vi "LockOut.vi"() -> ()   [LabVIEW 2019]
uses:
  <vilib>/NI/AMC/Read Termination Message.vi
  <vilib>/NI/AMC/Create Single Message.vi
  <vilib>/NI/AMC/Update Message Routing Info.vi
  <vilib>/NI/AMC/Globals.vi
  <vilib>/NI/AMC/Send Message.vi
  <vilib>/NI/AMC/AMC.lvlib
panel:
  out "By Emp:":string
  out "status":string
  in  "exit":bool
  # "Machine Locked Out"
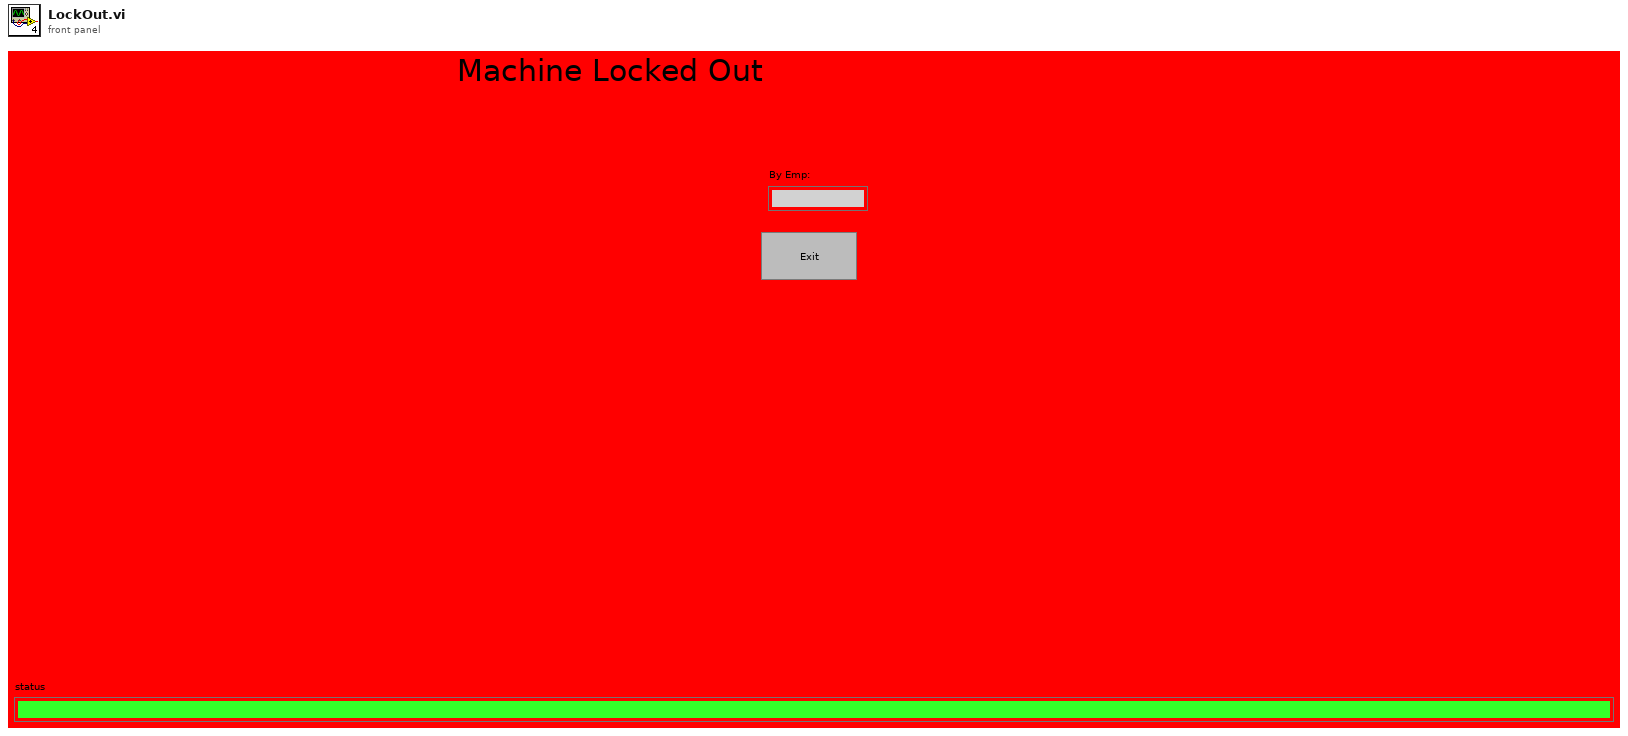
[diagram p1: front panel]
types:
  T1 = typedef "AMC.lvlib/Message Queue.ctl" = refnum<queue>
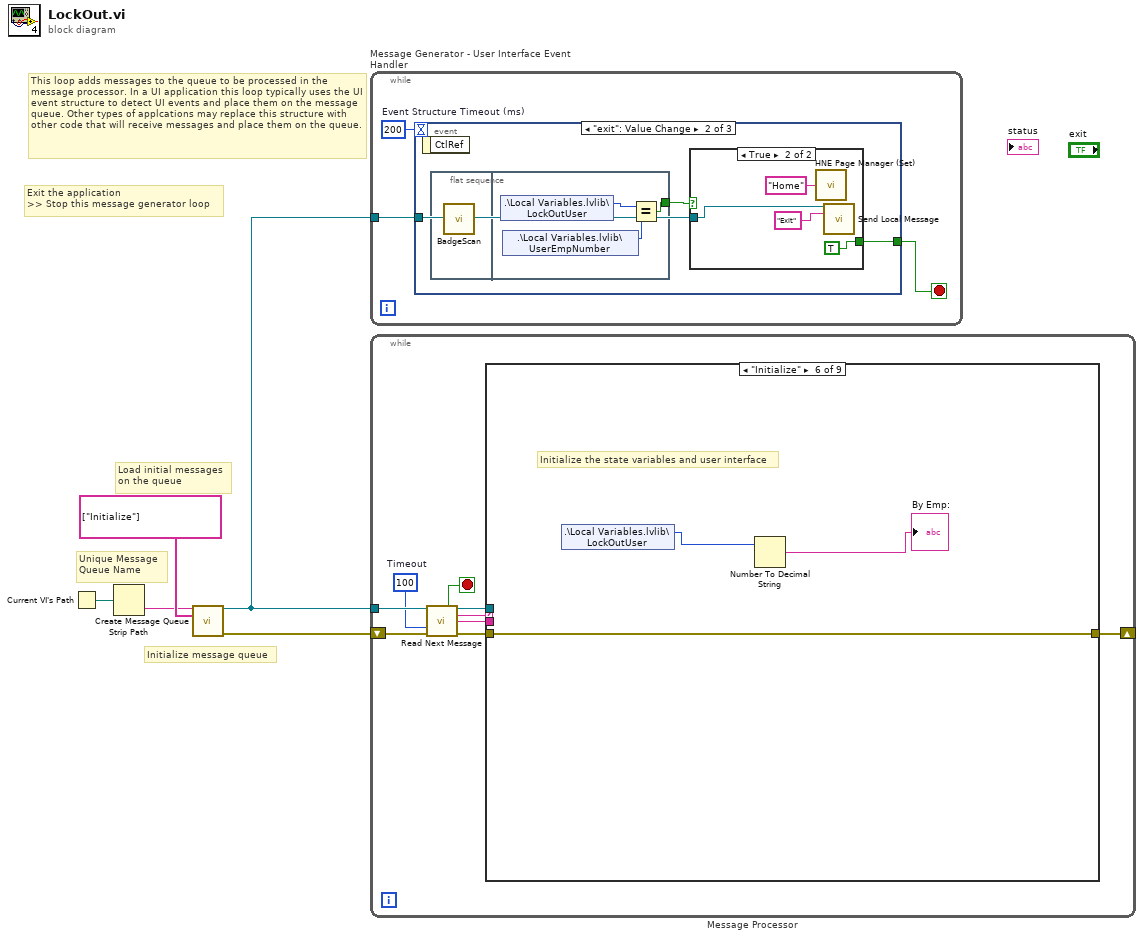
[diagram p0: block diagram]
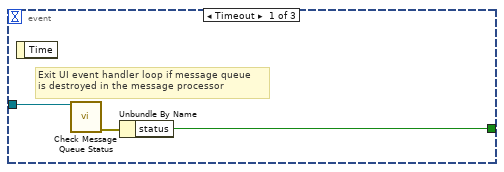
[diagram p2: hidden frame]
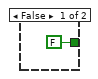
[diagram p3: hidden frame]
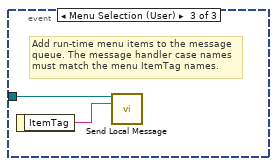
[diagram p4: hidden frame]
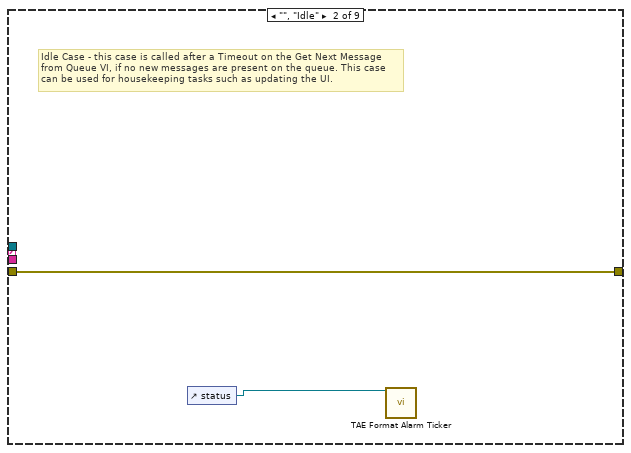
[diagram p6: hidden frame]
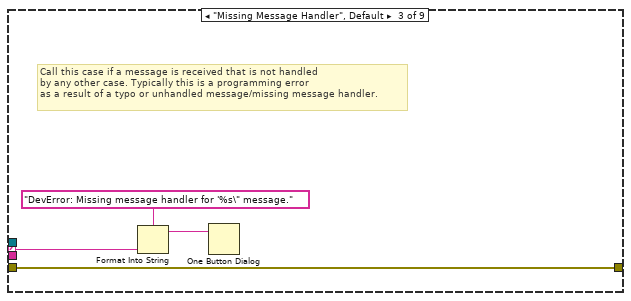
[diagram p7: hidden frame]
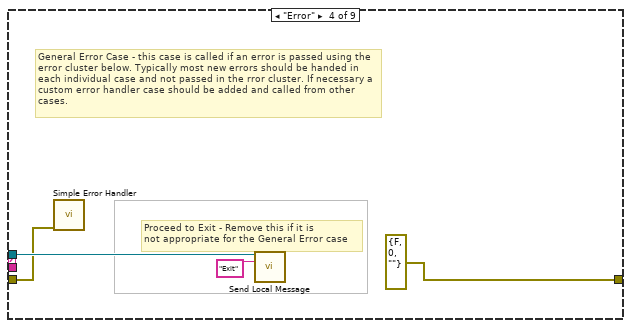
[diagram p8: hidden frame]
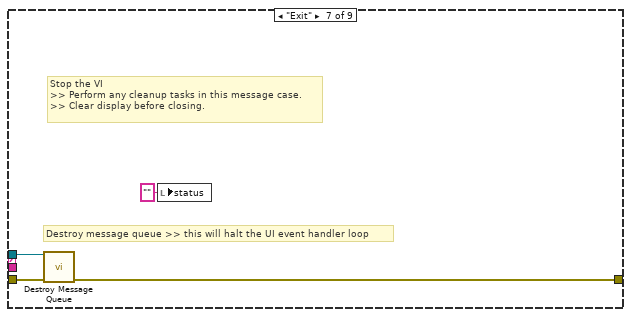
[diagram p10: hidden frame]
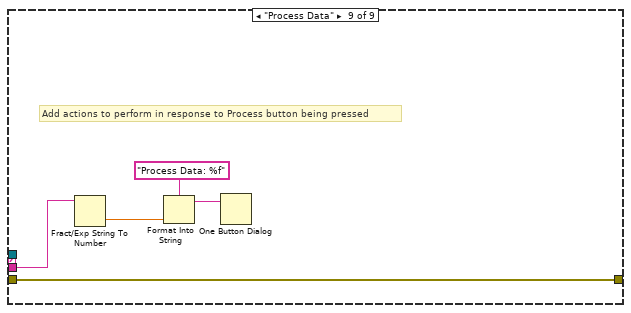
[diagram p12: hidden frame]
diagram:
  # "Exit the application\n>> Stop this message generator loop"
  # "This loop adds messages to the queue to be processed in the message processor. In a UI application this loop typically uses the UI event structure to detect UI events and place them on the message queue. Other types of applcations may replace this structure with other code that will receive messages and place them on the queue."
  # "Initialize message queue"
  # "Unique Message\nQueue Name"
  # "Load initial messages\non the queue"
  n1 = Current VI's Path() -> (path=w1:path)
  n2 = Strip Path(path=w1) -> (name=w4:string)  [unwired: 1 out]
  n3 = call <vilib>:"Create Message Queue.vi"("message queue name"=w4, "initial message names"=string[] ["Initialize"]) -> ("message queue out"=w3:T1, "error out"=w2:errorcluster)  [unwired: 12 in]
  n4 = while "Message Generator - User Interface Event Handler" {
    tunnel: w3 -> [w6]
    stop <- w7 stop-if-true
    w8 = 200  # Event Structure Timeout (ms)
    n5 = event shown="[1] \"exit\": Value Change" {
      selector: _ -> [_ _ _]
      dyn-events: _ -> [_ _ _]
      timeout: w8 -> [_ _ _]
      tunnel: [w9 w12 _] -> w7
      tunnel: w6 -> [w10 w14 w23]
      event Timeout {
        # "Exit UI event handler loop if message queue\nis destroyed in the message processor"
        n6 = event-data() -> ()  [unwired: 2 out]
        n7 = call <vilib>:"Check Message Queue Status.vi"("message queue in"=w10) -> ("error out"=w11:errorcluster)  [unwired: 10 in, 4 out]
        n8 = Unbundle By Name(w11) -> ("status"=w9:bool)
      }
      event "exit": Value Change {
        n9 = event-data() -> ()  [unwired: 2 out]
        n10 = flat-sequence {
          tunnel: [w15] -> w13
          frame #0 {
            n11 = call "BadgeScan.vi"() -> ()  [unwired: 11 in, 1 out]
          }
          frame #1 {
            n12 = shared-variable ".\\Local Variables.lvlib\\LockOutUser"() -> (w16:i32)  [unwired: 1 in, 1 out]
            n13 = shared-variable ".\\Local Variables.lvlib\\UserEmpNumber"() -> (w17:i32)  [unwired: 1 in, 1 out]
            n14 = Equal?(x=w16, y=w17) -> (x = y?=w15:bool)
          }
        }
        n15 = case shown="True" w13 {
          tunnel: w14 -> [_ w21]
          tunnel: [FALSE ("Discard?") TRUE ("Discard?")] -> w12
          frame False {
          }
          frame True {
            n16 = call <userlib>:"HNE Page Manager (Set).vi"("Next Page"="Home") -> ()  [unwired: 4 in, 1 out]
            n17 = call <vilib>:"Send Local Message.vi"("message queue in"=w21, "message name"="Exit") -> ()  [unwired: 11 in, 3 out]
          }
        }
      }
      event Menu Selection (User) {
        # "Add run-time menu items to the message\nqueue. The message handler case names must match the menu ItemTag names."
        n18 = event-data() -> ("ItemTag"=w24:string)  [unwired: 1 out]
        n19 = call <vilib>:"Send Local Message.vi"("message queue in"=w23, "message name"=w24) -> ()  [unwired: 11 in, 3 out]
      }
    }
  }
  n20 = while "Message Processor" {
    shift-left: w2 -> [w29]
    shift-right: [w33] -> _
    tunnel: w3 -> [w30]
    stop <- w32 stop-if-true
    w25 = 100  # Timeout
    n21 = call <vilib>:"Read Next Message.vi"("message queue in"=w30, "timeout (1 ms)"=w25, "error in"=w29) -> ("exit process?"=w32:bool, "message queue out"=w31:T1, "message name"=w27:string, "message value"=w26:string, "error out"=w28:errorcluster)  [unwired: 5 in, 3 out]
    n22 = case shown="\"Initialize\"" w27 {
      selector: w27 -> [_ _ w39 _ _ _ _ _ _]
      tunnel: w31 -> [_ _ _ w43 _ _ w50 _ _]
      tunnel: w28 -> [w34 w36 w40 w41 w45 w48 w51 w53 w58]
      tunnel: [w34 w36 w40 errorcluster {"status"=FALSE, "code"=0, "source"=""} ("error out") w45 w48 w49 w53 w58] -> w33
      tunnel: w26 -> [_ _ _ _ _ _ _ _ w57]
      frame "---------- Framework Operations ----------" {
        # "Dummy case to add a seperator in the Case Structure menu"
      }
      frame "", "Idle" {
        # "Idle Case - this case is called after a Timeout on the Get Next Message from Queue VI, if no new messages are present on the queue. This case can be used for housekeeping tasks such as updating the UI."
        n23 = control-ref of="status"() -> (w35:refnum<vi>)
        n24 = call <userlib>:"TAE Format Alarm Ticker.vi"("Alarm Ticker Ref"=w35) -> ()  [unwired: 15 in]
      }
      frame "Missing Message Handler", Default {
        # "Call this case if a message is received that is not handled \nby any other case. Typically this is a programming error\nas a result of a typo or unhandled message/missing message handler."
        n25 = Format Into String(format string="DevError: Missing message handler for '%s\" message." ("message"), w39) -> (resulting string=w37:string)  [unwired: 2 in, 1 out]
        n26 = One Button Dialog(message=w37) -> ()  [unwired: 2 out]
      }
      frame "Error" {
        # "Proceed to Exit - Remove this if it is\nnot appropriate for the General Error case"
        # "General Error Case - this case is called if an error is passed using the error cluster below. Typically most new errors should be handed in each individual case and not passed in the rror cluster. If necessary a custom error handler case should be added and called from other cases."
        n27 = call <vilib>:"Simple Error Handler.vi"("error in (no error)"=w41) -> ()  [unwired: 1 in, 8 out]
        n28 = call <vilib>:"Send Local Message.vi"("message queue in"=w43, "message name"="Exit") -> ()  [unwired: 11 in, 3 out]
      }
      frame "---------- Generic Operations ----------" {
        # "Dummy case to add a seperator in the Case Structure menu"
      }
      frame "Initialize" {
        # "Initialize the state variables and user interface"
        n29 = shared-variable ".\\Local Variables.lvlib\\LockOutUser"() -> (w47:i32)  [unwired: 1 in, 1 out]
        n30 = Number To Decimal String(number=w47) -> (decimal integer string=→"By Emp:":string)  [unwired: 1 in]
      }
      frame "Exit" {
        # "Destroy message queue >> this will halt the UI event handler loop"
        # "Stop the VI\n>> Perform any cleanup tasks in this message case.\n>> Clear display before closing."
        n31 = call <vilib>:"Destroy Message Queue.vi"("message queue in"=w50, "error in"=w51) -> ("error out"=w49:errorcluster)  [unwired: 11 in, 2 out]
        n32 = local write "status"("" ("Status")) -> ()
      }
      frame "---------- Application Operations ----------" {
        # "Dummy case to add a seperator in the Case Structure menu"
      }
      frame "Process Data" {
        # "Add actions to perform in response to Process button being pressed"
        n33 = Fract/Exp String To Number(string=w57) -> (number=w56:dbl)  [unwired: 4 out]
        n34 = Format Into String(format string="Process Data: %f" ("message"), w56) -> (resulting string=w54:string)  [unwired: 2 in, 1 out]
        n35 = One Button Dialog(message=w54) -> ()  [unwired: 2 out]
      }
    }
  }
